vi "Calculate rectangle.vi"(8 "error in (no error)":errorcluster, 10 "xyzs array":dbl[](array[numeric]), 11 "Tomo in":refnum<class "Tomo.lvclass">) -> (0 "error out":errorcluster, 3 "Tomo out":refnum<class "Tomo.lvclass">, 5 "rectangle":i32[](array[numeric]))   [LabVIEW 2012, in "Tomo.lvclass"]
uses:
  Tomo.lvclass
  Tomo.lvclass/Tomo.ctl
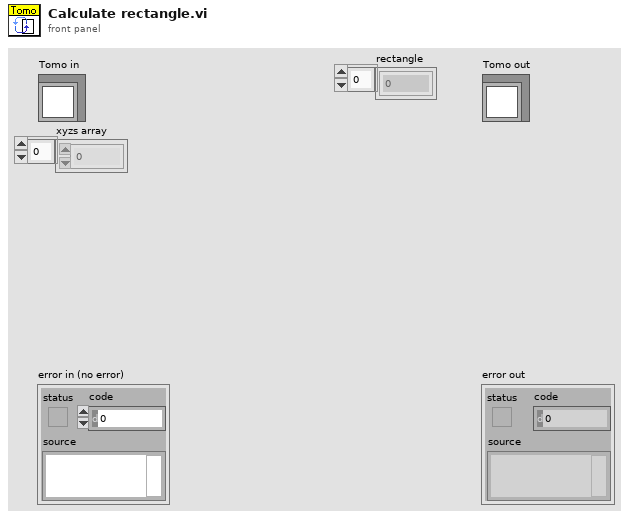
[diagram p1: front panel]
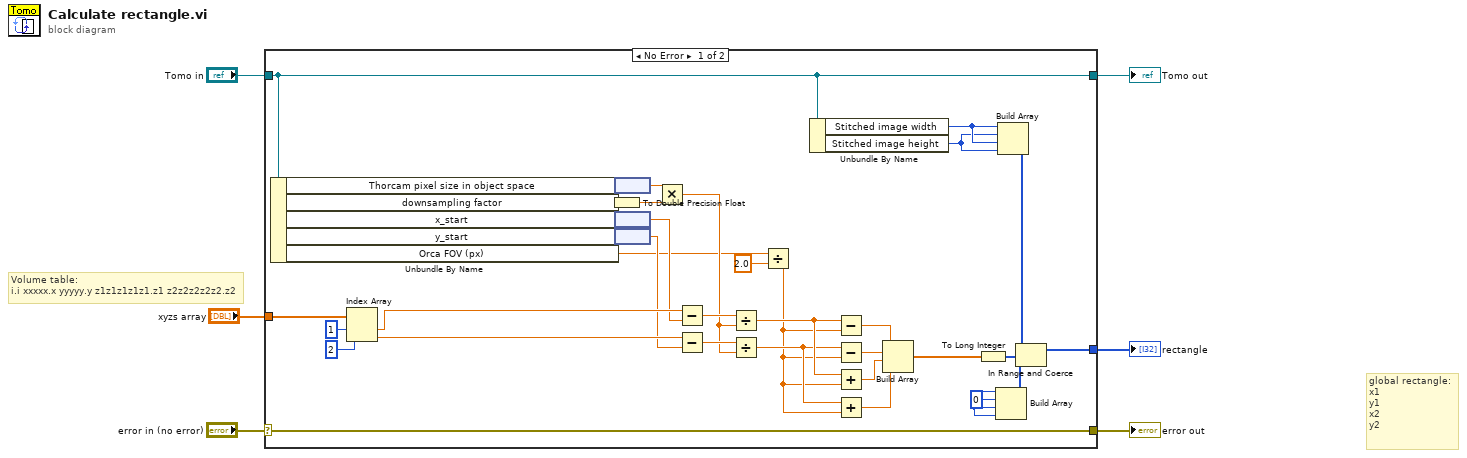
[diagram p0: block diagram]
diagram:
  # "Volume table: \ni.i xxxxx.x yyyyy.y z1z1z1z1z1.z1 z2z2z2z2z2.z2"
  # "global rectangle:\nx1\ny1\nx2\ny2"
  n1 = case shown="No Error" "error in (no error)" {
    selector: "error in (no error)" -> [w41 w43]
    tunnel: [w41 w43] -> w5
    tunnel: [w27 w42] -> w3
    tunnel: "Tomo in" -> [w27 w42]
    tunnel: "xyzs array" -> [w40 _]
    tunnel: [w20 _] -> w1
    frame No Error {
      w23 = 0 ("runtime cluster.Pretomo.Stitched image height")
      n2 = Unbundle By Name(w27) -> ("Thorcam pixel size in object space"=w29:dbl[unit], "downsampling factor"=w31:u32, "x_start"=w36:dbl[unit], "y_start"=w34:dbl[unit], "Orca FOV (px)"=w16:dbl)
      n3 = Index Array(array=w40, index #1=1 ("index"), index #2=2 ("index")) -> (element #1=w37:dbl, element #2=w33:dbl)
      n4 = To Double Precision Float(number=w31) -> (double precision float=w30:dbl)
      n5 = node(w29) -> (w28:dbl)
      n6 = node(w36) -> (w35:dbl)
      n7 = node(w34) -> (w32:dbl)
      n8 = Multiply(x=w28, y=w30) -> (x*y=w17:dbl)
      n9 = Subtract(x=w37, y=w35) -> (x-y=w19:dbl)
      n10 = Subtract(x=w33, y=w32) -> (x-y=w18:dbl)
      n11 = Divide(x=w19, y=w17) -> (x/y=w13:dbl)
      n12 = Divide(x=w18, y=w17) -> (x/y=w12:dbl)
      n13 = Divide(x=w16, y=2.0) -> (x/y=w11:dbl)
      n14 = Unbundle By Name(w27) -> ("Stitched image width"=w25:i32, "Stitched image height"=w24:i32)
      n15 = Subtract(x=w13, y=w11) -> (x-y=w14:dbl)
      n16 = Subtract(x=w12, y=w11) -> (x-y=w10:dbl)
      n17 = Add(x=w13, y=w11) -> (x+y=w9:dbl)
      n18 = Add(x=w12, y=w11) -> (x+y=w8:dbl)
      n19 = Build Array(w14, w10, w9, w8) -> (w7:dbl[])
      n20 = To Long Integer(number=w7) -> (32bit integer=w26:i32[])
      n21 = Build Array(w23, w23, w23, w23) -> (w22:i32[])
      n22 = Build Array(w25, w24, w25, w24) -> (w21:i32[])
      n23 = In Range and Coerce(upper limit=w21, x=w26, lower limit=w22) -> (coerced(x)=w20:i32[])  [unwired: 1 out]
    }
    frame Error {
    }
  }
  "error out" <- w5
  "Tomo out" <- w3
  "rectangle" <- w1
